vi "Process command line arguments.vi"(8 "error in (no error)":errorcluster, 10 "arguments":string[](array[string]), 11 "Murmex in":refnum<class "ServiceManager.lvclass">) -> (0 "error out":errorcluster, 3 "Murmex out":refnum<class "ServiceManager.lvclass">)   [LabVIEW 2012, in "ServiceManager.lvclass"]
doc: "If the EXE build of a component is started via the command line, its ID has to be handed over as a command line parameter: \nMyLittleComponent.exe id=John\n\nThis VI extracts the ID from the command line parameters and sets it if found."
uses:
  ServiceManager.lvclass
  Murmex/LabVIEW/Murmex/Murmex/Murmex.lvclass
panel:
  out "value":string
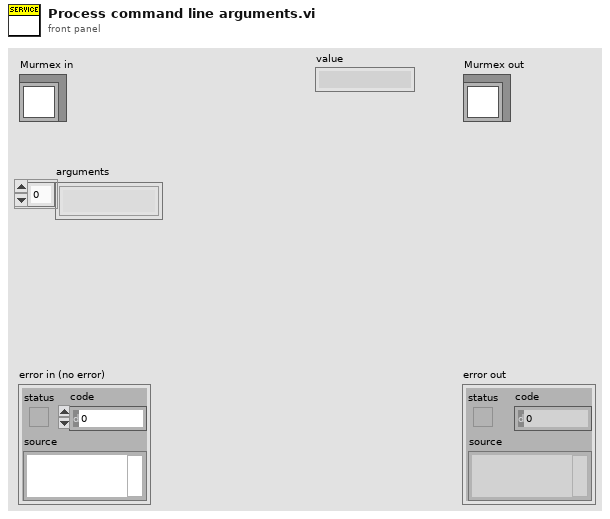
[diagram p1: front panel]
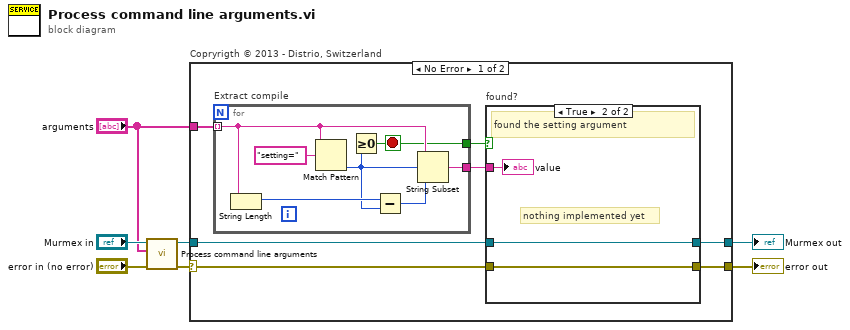
[diagram p0: block diagram]
diagram:
  n1 = call-parent "Process command line arguments.vi"("error in (no error)"="error in (no error)", "arguments"="arguments", "Murmex in"="Murmex in") -> ("error out"=w5:errorcluster, "Murmex out"=w2:refnum<class "ServiceManager.lvclass">)  [unwired: 7 in]
  n2 = case "Copryrigth © 2013 - Distrio, Switzerland" shown="No Error" w5 {
    selector: w5 -> [w9 w28]
    tunnel: [w8 w28] -> w4
    tunnel: [w11 w27] -> w3
    tunnel: w2 -> [w12 w27]
    tunnel: "arguments" -> [w14 _]
    frame No Error {
      n3 = for "Extract compile" {
        tunnel: w14 -> [w25] mode=indexing
        tunnel: [w22] -> w10
        tunnel: [w20] -> w13
        stop <- w20 stop-if-true
        n4 = String Length(string=w25) -> (length=w24:i32)
        n5 = Match Pattern(string=w25, regular expression="setting=") -> (offset past match=w21:i32)  [unwired: 1 in, 3 out]
        n6 = Greater Or Equal To 0?(x=w21) -> (x >= 0?=w20:bool)
        n7 = Subtract(x=w24, y=w21) -> (x-y=w23:i32)
        n8 = String Subset(string=w25, offset (0)=w21, length (rest)=w23) -> (substring=w22:string)
      }
      n9 = case "found?" shown="True" w13 {
        tunnel: w12 -> [w16 w19]
        tunnel: [w16 w19] -> w11
        tunnel: w10 -> [_ w17]
        tunnel: w9 -> [w15 w18]
        tunnel: [w15 w18] -> w8
        frame False {
        }
        frame True {
          # "nothing implemented yet"
          # "found the setting argument"
          "value" <- w17
        }
      }
    }
    frame Error {
    }
  }
  "error out" <- w4
  "Murmex out" <- w3
